vi "parse_from_rio.vi"(4 "Error In":errorcluster, 7 "msg in":string) -> (0 "Error Out":errorcluster, 2 "from_rio":cluster{"speed_is":dbl, "steering_is":dbl}, 3 "msg out":string)   [LabVIEW 2016]
uses:
  <userlib>/ROS for LabVIEW Software/ROS/MessageParsing/std_msgs/subs/parse_float64_scalar.vi
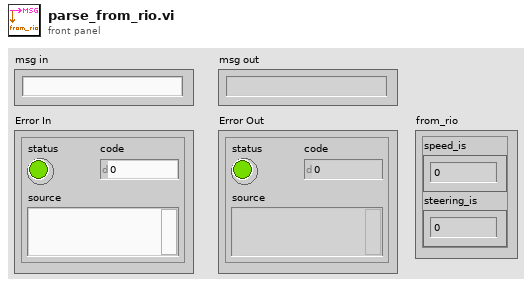
[diagram p1: front panel]
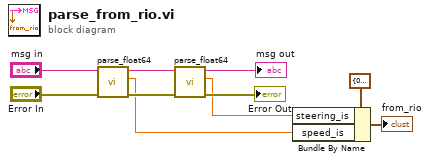
[diagram p0: block diagram]
diagram:
  n1 = call-poly <userlib>:"parse_float64.vi"("error in"="Error In", "msg in"="msg in") -> ("error out"=w10:errorcluster, "number"=w1:dbl, "msg out"=w9:string)  [unwired: 3 in]
  n2 = call-poly <userlib>:"parse_float64.vi"("error in"=w10, "msg in"=w9) -> ("error out"=→"Error Out":errorcluster, "number"=w2:dbl, "msg out"=→"msg out":string)  [unwired: 3 in]
  n3 = Bundle By Name(cluster=cluster{"speed_is":dbl, "steering_is":dbl} {"speed_is"=0.0, "steering_is"=0.0}, "steering_is"=w2, "speed_is"=w1) -> (→"from_rio":cluster{"speed_is":dbl, "steering_is":dbl})
